vi "Read_Excel_Values.vi"() -> ()   [LabVIEW 2017]
doc: "This simple program is a demonstration of how to use the LabVIEW Report Generation Toolkit to read data from Excel."
uses:
  <vilib>/addons/_office/excel.llb/Excel Get Data ([dbl]).vi
  <vilib>/addons/_office/excel.llb/Excel Get Data ([str]).vi
  <vilib>/addons/_office/excel.llb/Excel Get Data (i32).vi
  <vilib>/Utility/NIReport.llb/NI_report.lvclass
  <vilib>/Utility/NIReport.llb/Excel/NI_Excel.lvclass
  <vilib>/addons/_office/NI_ReportGenerationToolkit.lvlib
panel:
  out "Sheet 3 Data":i32
  out "Sheet 2 Data":string[][](array[string])
  out "Sheet 1 Data":dbl[][](array[numeric])
  # "Overview: This simple program is a demonstration of how to use the LabVIEW Report Generation Toolkit to read data from Excel.\nRequirements: LabVIEW 2012 (or compatible), LabVIEW Report Generation Toolkit 2012 (or compatible)\nInstructions:\n1. Run the VI\n2. You will be prompted to enter the location for the excel file, browse for the the excel file located in the same directory of this VI\n3. Click OK"
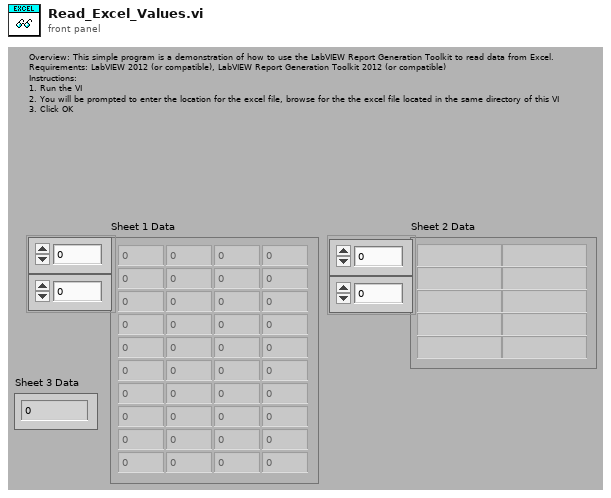
[diagram p1: front panel]
types:
  T1 = enum16{"Standard Report", "HTML", "Word", "Excel"}
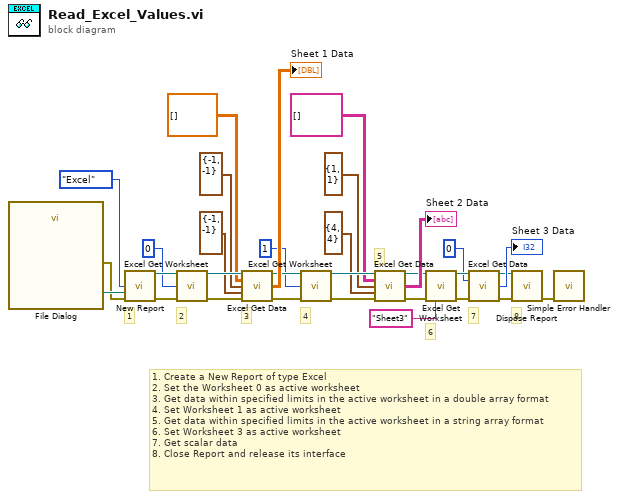
[diagram p0: block diagram]
diagram:
  # "1. Create a New Report of type Excel\n2. Set the Worksheet 0 as active worksheet\n3. Get data within specified limits in the active worksheet in a double array format\n4. Set Worksheet 1 as active worksheet\n5. Get data within specified limits in the active worksheet in a string array format \n6. Set Worksheet 3 as active worksheet\n7. Get scalar data \n8. Close Report and release its interface"
  # "8"
  # "7"
  # "6"
  # "5"
  # "4"
  # "3"
  # "2"
  # "1"
  n1 = call "File Dialog"() -> ("selected path"=w11:path, "error out"=w1:errorcluster)  [unwired: 7 in, 7 out]
  n2 = call <vilib>:"New Report.vi"("report type"=T1."Excel", "template (empty)"=w11, "error in (no error)"=w1) -> ("report out"=w31:refnum<class "NI_report.lvclass">, "error out"=w22:errorcluster)  [unwired: 3 in, 8 out]
  n3 = call <vilib>:"Excel Get Worksheet.vi"("report in"=w31, "worksheet index (0)"=0, "error in (no error)"=w22) -> ("report out"=w30:refnum<class "NI_report.lvclass">, "error out"=w21:errorcluster)  [unwired: 11 out]
  n4 = call-poly <vilib>:"Excel Get Data.vi"("report in"=w30, "data type"=dbl[][] [], "start (-1, -1)"=cluster{"row":i32, "column":i32} {"row"=-1, "column"=-1}, "end (-1, -1)"=cluster{"row":i32, "column":i32} {"row"=-1, "column"=-1}, "error in (no error)"=w21) -> ("report out"=w25:refnum<class "NI_report.lvclass">, "data"=→"Sheet 1 Data":dbl[][], "error out"=w17:errorcluster)  [unwired: 8 out]
  n5 = call <vilib>:"Excel Get Worksheet.vi"("report in"=w25, "worksheet index (0)"=1, "error in (no error)"=w17) -> ("report out"=w23:refnum<class "NI_report.lvclass">, "error out"=w16:errorcluster)  [unwired: 11 out]
  n6 = call-poly <vilib>:"Excel Get Data.vi"("report in"=w23, "data type"=string[][] [], "start (-1, -1)"=cluster{"row":i32, "column":i32} {"row"=1, "column"=1}, "end (-1, -1)"=cluster{"row":i32, "column":i32} {"row"=4, "column"=4}, "error in (no error)"=w16) -> ("report out"=w8:refnum<class "NI_report.lvclass">, "data"=→"Sheet 2 Data":string[][], "error out"=w6:errorcluster)  [unwired: 8 out]
  n7 = call <vilib>:"Excel Get Worksheet.vi"("report in"=w8, "error in (no error)"=w6, "name (\"\")"="Sheet3" ("name (\"\")")) -> ("report out"=w9:refnum<class "NI_report.lvclass">, "error out"=w10:errorcluster)  [unwired: 1 in, 10 out]
  n8 = call-poly <vilib>:"Excel Get Data.vi"("report in"=w9, "data type"=0, "error in (no error)"=w10) -> ("report out"=w2:refnum<class "NI_report.lvclass">, "data"=→"Sheet 3 Data":i32, "error out"=w7:errorcluster)  [unwired: 1 in, 9 out]
  n9 = call-dynamic "Dispose Report.vi"("report in"=w2, "error in (no error)"=w7) -> ("error out"=w18:errorcluster)  [unwired: 3 in, 10 out]
  n10 = call <vilib>:"Simple Error Handler.vi"("error in (no error)"=w18) -> ()  [unwired: 4 in, 5 out]
